vi "Fi_delta.vi"(8 "input valid":bool=TRUE, 10 "Fi_delta":fxp<+/-,32,4>, 11 "Fi_start":fxp<+/-,32,4>) -> (0 "output valid":bool, 3 "Fi out":fxp<+/-,32,4>)   [LabVIEW 2013]
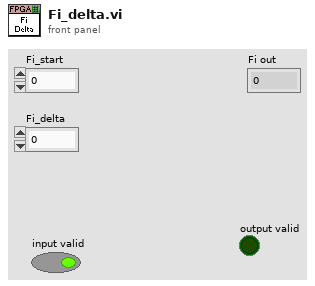
[diagram p1: front panel]
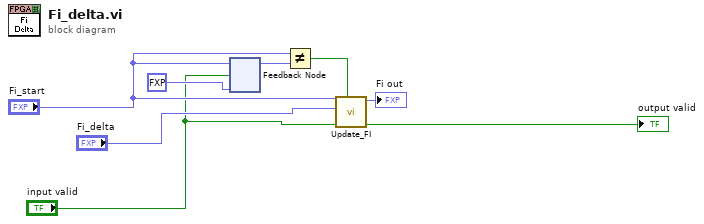
[diagram p0: block diagram]
diagram:
  n1 = feedback #1(fxp<+/-,32,4> -1.0 ("Fi_start")) -> (w7:fxp<+/-,32,4>)
  n2 = feedback-in #1("Fi_start", "input valid") -> ()
  n3 = Not Equal?(x="Fi_start", y=w7) -> (x != y?=w5:bool)
  n4 = call "Update_FI.vi"("Reset"=w5, "input valid"="input valid", "Fi_delta"="Fi_delta", "Fi_start"="Fi_start") -> ("output valid"=→"output valid":bool, "Fi out"=→"Fi out":fxp<+/-,32,4>)  [unwired: 6 in]
